vi "Open File.vi"(8 "error in (no error)":errorcluster, 11 "Spectrum Recorder in":refnum<class "Spectrum Recorder.lvclass">) -> (0 "error out":errorcluster, 3 "Spectrum Recorder out":refnum<class "Spectrum Recorder.lvclass">)   [LabVIEW 2016, in "Spectrum Recorder.lvclass"]
uses:
  Spectrum Recorder.lvclass
  NHMFL_Core/Libraries/File/Controls/File formats.ctl
  Spectrum Recorder.lvclass/Spectrum Recorder.ctl
  Read Spectrum Recorder Configuration.vi
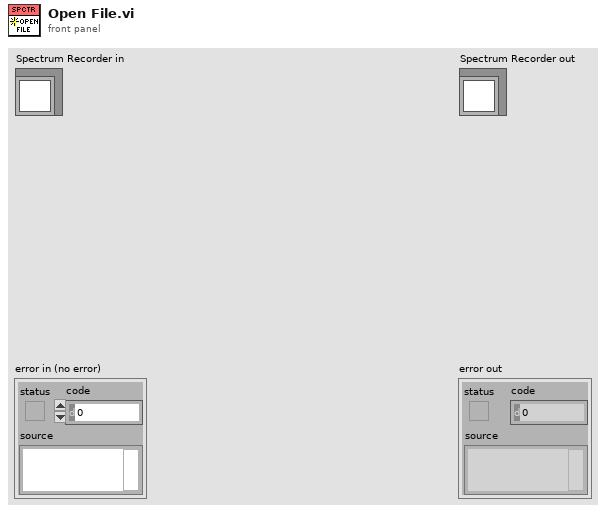
[diagram p1: front panel]
types:
  T1 = enum16{"open", "open or create", "create or replace", "create", "open (read-only)"}
  T2 = typedef "File formats.ctl" = enum16{"TDMS", "ASCII", "BINARY"}
  T3 = typedef "Spectrum Recorder Configuration.ctl" = cluster{"Start":dbl, "End":dbl, "Duration":dbl, "Filter time constant":dbl, "Repeat (-1: forever)":i32, "Update rate":dbl, "Data storage folder":path}
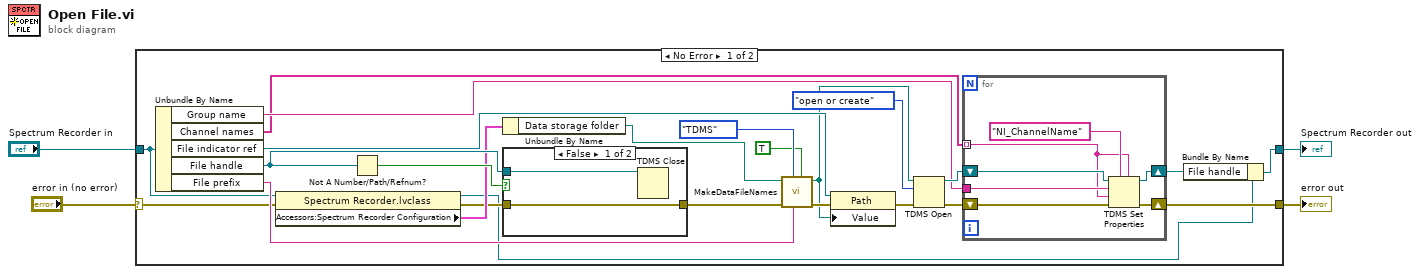
[diagram p0: block diagram]
diagram:
  n1 = case shown="No Error" "error in (no error)" {
    selector: "error in (no error)" -> [w8 w40]
    tunnel: [w11 w40] -> w3
    tunnel: [w21 w39] -> w1
    tunnel: "Spectrum Recorder in" -> [w6 w39]
    frame No Error {
      n2 = Unbundle By Name(w6) -> ("Group name"=w14:string, "Channel names"=w13:string[], "File indicator ref"=w19:refnum<vi>, "File handle"=w27:refnum<k34>, "File prefix"=w17:string)
      n3 = property class="Spectrum Recorder.lvclass"(reference=w6, error in=w8) -> (reference out=w5:refnum<class "Spectrum Recorder.lvclass">, error out=w7:errorcluster, "Accessors:Spectrum Recorder Configuration"=w10:T3)
      n4 = Not A Number/Path/Refnum?(number/path/refnum=w27) -> (NaN/Path/Refnum?=w28:bool)
      n5 = Unbundle By Name(w10) -> ("Data storage folder"=w9:path)
      n6 = case shown="False" w28 {
        tunnel: w27 -> [w37 _]
        tunnel: w7 -> [w36 w38]
        tunnel: [w36 w38] -> w26
        frame False {
          n7 = TDMS Close(11:w37) -> ()  [unwired: 1 in, 2 out]
        }
        frame True {
        }
      }
      n8 = call "MakeDataFileNames.vi"("Include time"=TRUE, "File Prefix"=w17, "File format"=File_formats."TDMS", "Error In"=w26, "Root Data Folder"=w9) -> ("Error Out"=w24:errorcluster, "Data File  Path"=w18:path)  [unwired: 3 in, 2 out]
      n9 = property class="Path"(reference=w19, error in=w24, "Value"=w18) -> (error out=w20:errorcluster)  [unwired: 1 out]
      n10 = TDMS Open(8:w20, 10:T1."open or create" ("operation (0:open)"), 11:w18) -> (0:w12:errorcluster, 3:w16:refnum<k34>)  [unwired: 4 in]
      n11 = for {
        tunnel: w14 -> [w33]
        tunnel: w13 -> [w29] mode=indexing
        shift-right: [w34] -> w15
        shift-left: w16 -> [w35]
        shift-right: [w31] -> w11
        shift-left: w12 -> [w32]
        n12 = TDMS Set Properties(5:w29, 7:"NI_ChannelName", 8:w32, 9:w29, 10:w33, 11:w35) -> (0:w31:errorcluster, 3:w34:refnum<k34>)  [unwired: 2 out]
      }
      n13 = Bundle By Name(cluster=w5, "File handle"=w15) -> (w21:refnum<class "Spectrum Recorder.lvclass">)
    }
    frame Error {
    }
  }
  "error out" <- w3
  "Spectrum Recorder out" <- w1
